vi "ex_Loop Overhead.vi"(2 "Bottom Button Bar":cluster{"Ok":bool, "Cancel":bool, "Help":bool}, 4 "No Delay":bool, 5 "Help string to search for":string="Reference Curve") -> (0 "Loop Terminator":bool, 1 "Data Valid":bool)   [LabVIEW 2017]
doc: "Handles the Bottom Button Bar (OK, Cancel, Help) passed in for a calling VI. Data Valid is set to TRUE if the OK button is pressed. The Loop Terminator is set to TRUE if either the OK or Cancel buttons are pressed. Opens the online help manuals to the appropriate location when the Help button is pressed.\n\nUnless the No Delay value is TRUE, the panel of the calling VI is opened the second time this VI is run. After the first run, a 50 ms timer is also run for each subsequent iteration.\n\nAn alternate way to handle the bottom button bar is to use an event structure and look for the OK, Cancel, or Help button value changes."
panel:
  in  "Second Time":bool=TRUE
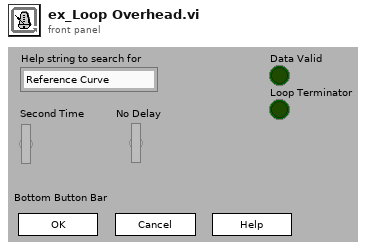
[diagram p1: front panel]
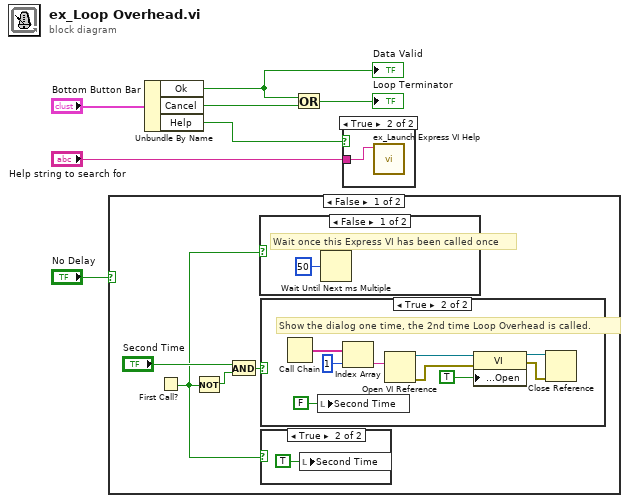
[diagram p0: block diagram]
diagram:
  n1 = case shown="False" "No Delay" {
    frame False {
      n2 = First Call?() -> (First Call?: T/F=w8:bool)
      n3 = Not(x=w8) -> (.not. x?=w11:bool)
      n4 = And(x="Second Time", y=w11) -> (x .and. y?=w10:bool)
      n5 = case shown="False" w8 {
        frame False {
          # "Wait once this Express VI has been called once"
          n6 = Wait Until Next ms Multiple(millisecond multiple=u32 50 ("milliseconds to wait")) -> ()  [unwired: 1 out]
        }
        frame True {
        }
      }
      n7 = case shown="True" w10 {
        frame False {
        }
        frame True {
          # "Show the dialog one time, the 2nd time Loop Overhead is called."
          n8 = Call Chain() -> (call chain=w20:string[])
          n9 = local write "Second Time"(FALSE ("Second Time")) -> ()
          n10 = Index Array(array=w20, index=1 ("Index")) -> (element=w18:string)
          n11 = Open VI Reference(vi path=w18) -> (vi reference=w16:refnum<vi>, error out=w17:errorcluster)  [unwired: 5 in]
          n12 = property class="VI"(reference=w16, error in=w17, "Front Panel Window:Open"=TRUE) -> (reference out=w15:refnum<vi>, error out=w14:errorcluster)
          n13 = Close Reference(reference=w15, error in (no error)=w14) -> ()  [unwired: 1 out]
        }
      }
      n14 = case shown="True" w8 {
        frame False {
        }
        frame True {
          n15 = local write "Second Time"(TRUE ("Second Time")) -> ()
        }
      }
    }
    frame True {
    }
  }
  n16 = Unbundle By Name("Bottom Button Bar") -> ("Ok"=w6:bool, "Cancel"=w5:bool, "Help"=w7:bool)
  "Data Valid" <- w6
  n17 = Or(x=w6, y=w5) -> (x .or. y?=→"Loop Terminator":bool)
  n18 = case shown="True" w7 {
    tunnel: "Help string to search for" -> [_ w23]
    frame False {
    }
    frame True {
      n19 = call <vilib>:"ex_Launch Express VI Help.vi"("Keyword/HTML File"=w23) -> ()  [unwired: 6 in, 1 out]
    }
  }
